vi "Message Check.vi"(8 "error in (no error)":errorcluster, 10 "Message Payload":T1, 11 "Button Object Array In":refnum<class "Button.lvclass">[](array[class])) -> (0 "error out":errorcluster, 3 "Button Object Array Out":refnum<class "Button.lvclass">[](array[class]))   [LabVIEW 2019]
doc: "This VI will go through all messages in the Queue. A message payload contains the Button ID and the Current time."
uses:
  Button Class/Button.lvclass
  Button Class/TCP Message Payload.ctl
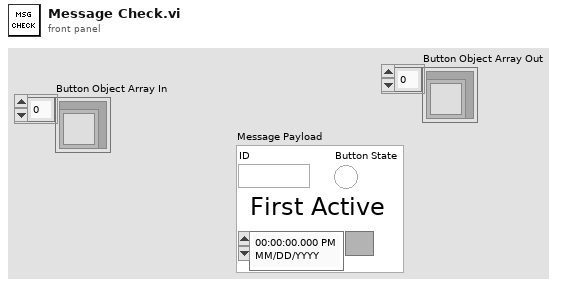
[diagram p1: front panel]
types:
  T1 = typedef "TCP Message Payload.ctl" = cluster{"ID":string, "First Active":timestamp, "Button State":bool}
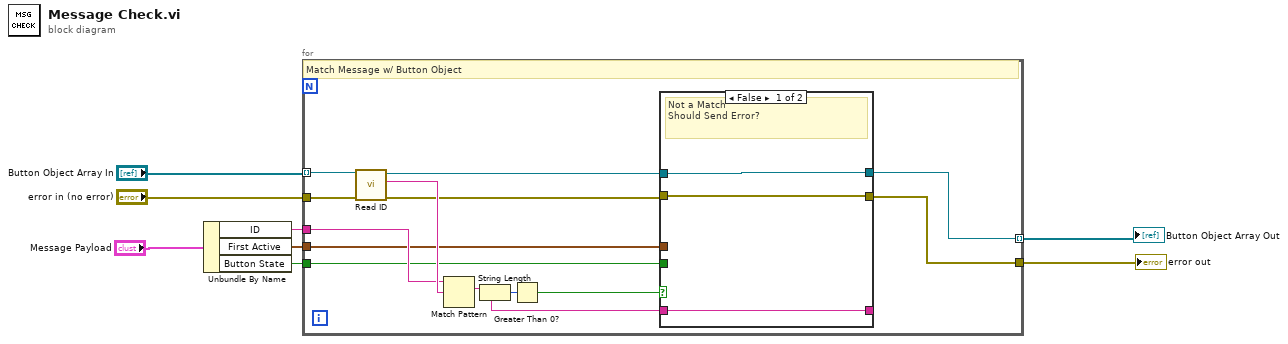
[diagram p0: block diagram]
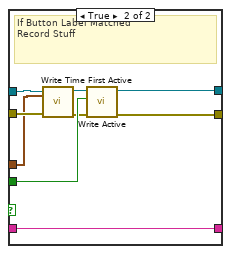
[diagram p2: hidden frame]
diagram:
  n1 = Unbundle By Name("Message Payload") -> ("ID"=w4:string, "First Active"=w3:timestamp, "Button State"=w2:bool)
  n2 = for {
    tunnel: "Button Object Array In" -> [w21] mode=indexing
    tunnel: w4 -> [w18]
    tunnel: w3 -> [w10]
    tunnel: [w14] -> w8
    tunnel: "error in (no error)" -> [w20]
    tunnel: [w12] -> w5 mode=indexing
    tunnel: w2 -> [w11]
    # "Match Message w/ Button Object"
    n3 = call-dynamic "Read ID.vi"("error in (no error)"=w20, "Button in"=w21) -> ("error out"=w15:errorcluster, "ID"=w19:string, "Button out"=w16:refnum<class "Button.lvclass">)  [unwired: 7 in]
    n4 = Match Pattern(string=w18, regular expression=w19) -> (match substring=w9:string)  [unwired: 1 in, 3 out]
    n5 = String Length(string=w9) -> (length=w17:i32)
    n6 = Greater Than 0?(x=w17) -> (x > 0?=w13:bool)
    n7 = case shown="False" w13 {
      tunnel: w16 -> [w23 w30]
      tunnel: w15 -> [w24 w32]
      tunnel: w10 -> [_ w29]
      tunnel: [w24 w26] -> w14
      tunnel: [w23 w27] -> w12
      tunnel: w11 -> [_ w33]
      tunnel: w9 -> [w22 w25]
      tunnel: [w22 w25] -> _
      frame False {
        # "Not a Match\nShould Send Error?"
      }
      frame True {
        # "If Button Label Matched\nRecord Stuff"
        n8 = call-dynamic "Write Time First Active.vi"("error in (no error)"=w32, "Time First Active"=w29, "Button in"=w30) -> ("error out"=w31:errorcluster, "Button out"=w28:refnum<class "Button.lvclass">)  [unwired: 7 in]
        n9 = call-dynamic "Write Active.vi"("error in (no error)"=w31, "Active"=w33, "Button in"=w28) -> ("error out"=w26:errorcluster, "Button out"=w27:refnum<class "Button.lvclass">)  [unwired: 7 in]
      }
    }
  }
  "error out" <- w8
  "Button Object Array Out" <- w5
